vi "pmu_Build Time Quality.vi"(0 "reported GPS information":T1, 1 "max time error [s]":dbl=1e-07 format="%#_15f", 9 "system info in":refnum<class "PMU System Info.lvclass">, 11 "error in (no error)":errorcluster) -> (4 "reporting timing information":T2 {"time quality flag" format="%.0b"}, 10 "system info out":refnum<class "PMU System Info.lvclass">, 15 "error out":errorcluster)   [LabVIEW 2011, in "NI_EP_PMU.lvlib"]
doc: "Outputs time quality flag bits, according to IEEE Std C37.118."
uses:
  <vilib>/addons/Electrical Power/PMU/Common/Controls/pmu_Reporting Time Information.ctl
  <vilib>/addons/Electrical Power/PMU/Common/Classes/PMU System Info/PMU System Info.lvclass
  <vilib>/addons/Electrical Power/PMU/Common/Controls/pmu_GPS Info.ctl
  <vilib>/addons/Electrical Power/PMU/NI_EP_PMU.lvlib
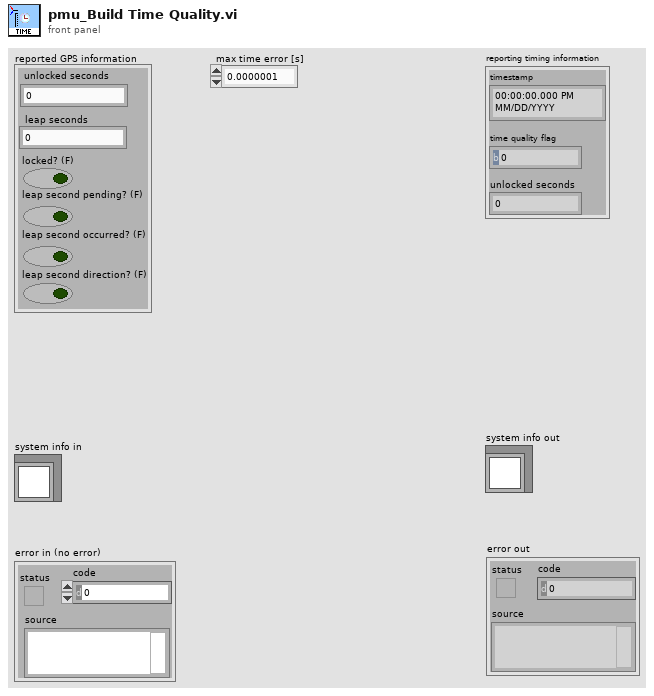
[diagram p1: front panel]
types:
  T1 = typedef "NI_EP_PMU.lvlib/pmu_GPS Info.ctl" = cluster{"unlocked seconds":u32, "leap seconds":i8, "locked? (F)":bool, "leap second pending? (F)":bool, "leap second occurred? (F)":bool, "leap second direction? (F)":bool}
  T2 = typedef "NI_EP_PMU.lvlib/pmu_Reporting Time Information.ctl" = cluster{"time quality flag":u8, "unlocked seconds":u32, "timestamp":timestamp}
  T3 = typedef "LVDateTimeRec.ctl" = cluster{"fractional second":dbl, "second":i32, "minute":i32, "hour":i32, "day of month":i32, "month":i32, "year":i32, "day of week":i32, "day of year":i32, "DST":i32}
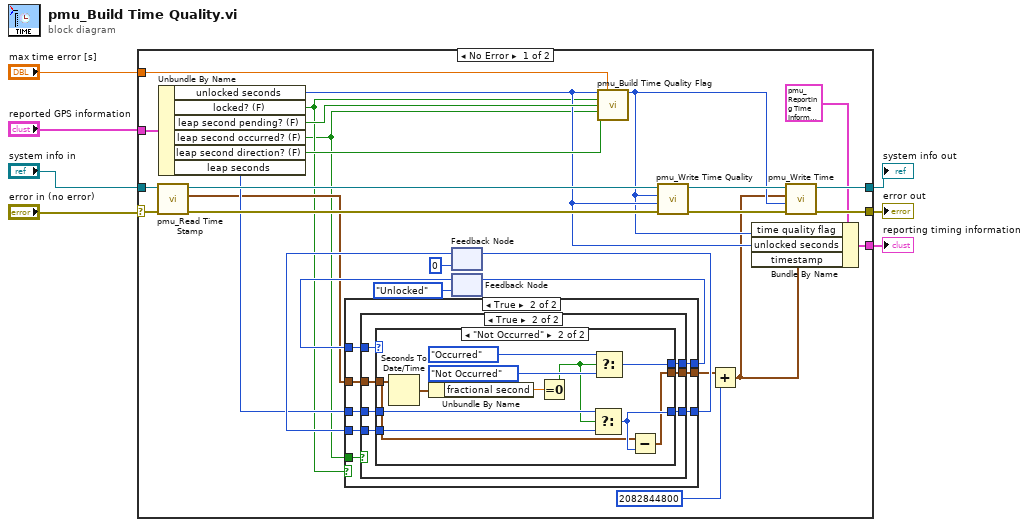
[diagram p0: block diagram]
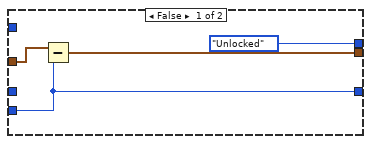
[diagram p2: hidden frame]
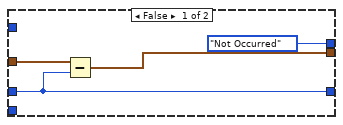
[diagram p3: hidden frame]
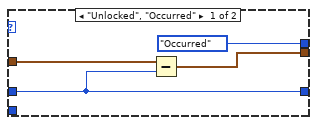
[diagram p4: hidden frame]
diagram:
  n1 = case shown="No Error" "error in (no error)" {
    selector: "error in (no error)" -> [w26 w75]
    tunnel: "system info in" -> [w27 _]
    tunnel: "max time error [s]" -> [w34 _]
    tunnel: [w32 w75] -> w6
    tunnel: [w31 _] -> w5
    tunnel: "reported GPS information" -> [w25 _]
    tunnel: [w21 _] -> w1
    frame No Error {
      n2 = call <vilib>:"pmu_Read Time Stamp.vi"("error in (no error)"=w26, "system info in"=w27) -> ("error out"=w28:errorcluster, "time stamp"=w14:timestamp, "system info out"=w29:refnum<class "PMU System Info.lvclass">)  [unwired: 7 in]
      n3 = Unbundle By Name(w25) -> ("unlocked seconds"=w23:u32, "locked? (F)"=w13:bool, "leap second pending? (F)"=w36:bool, "leap second occurred? (F)"=w8:bool, "leap second direction? (F)"=w35:bool, "leap seconds"=w15:i8)
      n4 = feedback #1(i8 0 ("leap seconds")) -> (w19:i8)
      n5 = feedback #2(enum16{"Unlocked", "Not Occurred", "Occurred"}."Unlocked" ("f")) -> (w17:enum16{"Unlocked", "Not Occurred", "Occurred"})
      n6 = case shown="True" w13 {
        tunnel: w14 -> [w40 w47]
        tunnel: w15 -> [_ w45]
        tunnel: w8 -> [_ w48]
        tunnel: [w38 w46] -> w12
        tunnel: [w39 w42] -> w20
        tunnel: w19 -> [w39 w41]
        tunnel: w17 -> [_ w43]
        tunnel: [enum16{"Unlocked", "Not Occurred", "Occurred"}."Unlocked" w44] -> w16
        frame False {
          n7 = Subtract(x=w40, y=w39) -> (x-y=w38:timestamp)
        }
        frame True {
          n8 = case shown="True" w48 {
            tunnel: w47 -> [w52 w54]
            tunnel: w45 -> [w50 w58]
            tunnel: [w51 w55] -> w46
            tunnel: [enum16{"Unlocked", "Not Occurred", "Occurred"}."Not Occurred" w59] -> w44
            tunnel: w43 -> [_ w53]
            tunnel: [w50 w56] -> w42
            tunnel: w41 -> [_ w57]
            frame False {
              n9 = Subtract(x=w52, y=w50) -> (x-y=w51:timestamp)
            }
            frame True {
              n10 = case shown="\"Not Occurred\"" w53 {
                tunnel: [enum16{"Unlocked", "Not Occurred", "Occurred"}."Occurred" w66] -> w59
                tunnel: w58 -> [w61 w72]
                tunnel: w57 -> [_ w71]
                tunnel: [w61 w70] -> w56
                tunnel: [w62 w69] -> w55
                tunnel: w54 -> [w63 w68]
                frame "Unlocked", "Occurred" {
                  n11 = Subtract(x=w63, y=w61) -> (x-y=w62:timestamp)
                }
                frame "Not Occurred" {
                  n12 = Seconds To Date/Time(time stamp (now)=w68) -> (date time rec=w74:T3)  [unwired: 1 in]
                  n13 = Unbundle By Name(w74) -> ("fractional second"=w73:dbl)
                  n14 = Equal To 0?(x=w73) -> (x = 0?=w64:bool)
                  n15 = Select(t=w72, s=w64, f=w71) -> (s? t:f=w70:i8)
                  n16 = Select(t=enum16{"Unlocked", "Not Occurred", "Occurred"}."Occurred", s=w64, f=enum16{"Unlocked", "Not Occurred", "Occurred"}."Not Occurred") -> (s? t:f=w66:enum16{"Unlocked", "Not Occurred", "Occurred"})
                  n17 = Subtract(x=w68, y=w70) -> (x-y=w69:timestamp)
                }
              }
            }
          }
        }
      }
      n18 = feedback-in #1(w20) -> ()
      n19 = feedback-in #2(w16) -> ()
      n20 = call <vilib>:"pmu_Build Time Quality Flag.vi"("unlocked seconds"=w23, "max time error per second (s)"=w34, "locked?"=w13, "leap second pending"=w36, "leap second occurred"=w8, "leap second direction"=w35) -> ("time quality flag"=w22:u8)  [unwired: 9 in]
      n21 = call <vilib>:"pmu_Write Time Quality.vi"("error in (no error)"=w28, "unlocked time"=w23, "time quality flag"=w22, "system info in"=w29) -> ("error out"=w33:errorcluster, "system info out"=w30:refnum<class "PMU System Info.lvclass">)  [unwired: 6 in]
      n22 = Add(x=w12, y=u32 2082844800 ("unsigned 32bit integer")) -> (x+y=w10:timestamp)
      n23 = Bundle By Name(cluster=T2 {"time quality flag"=0, "unlocked seconds"=0, "timestamp"=timestamp(0 s since 1904-01-01)} ("reporting timing information"), "time quality flag"=w22, "unlocked seconds"=w23, "timestamp"=w10) -> (w21:T2)
      n24 = call <vilib>:"pmu_Write Time .vi"("error in (no error)"=w33, "time quality"=w22, "time stamp"=w10, "system info in"=w30) -> ("error out"=w32:errorcluster, "system info out"=w31:refnum<class "PMU System Info.lvclass">)  [unwired: 6 in]
    }
    frame Error {
    }
  }
  "reporting timing information" <- w1
  "error out" <- w6
  "system info out" <- w5
